vi "set_IMAQdxSession.vi"(3 "error in (no error)":errorcluster, 4 "IMAQdx Session":T1, 5 "HGF_ImaqDx in":refnum<class "HGF_ImaqDx.lvclass">) -> (0 "error out":errorcluster, 2 "HGF_ImaqDx out":refnum<class "HGF_ImaqDx.lvclass">)   [LabVIEW 2014, in "HGF_IMAQ.lvlib" / "HGF_ImaqDx.lvclass"]
doc: "Set member: IMAQdx Session."
uses:
  HGF_ImaqDx.lvclass
  <vilib>/userdefined/High Color/IMAQdx.ctl
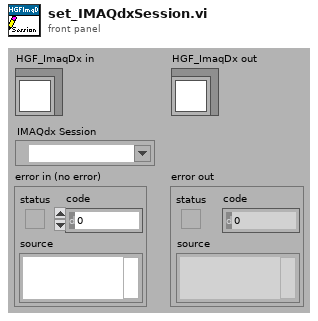
[diagram p1: front panel]
types:
  T1 = typedef "IMAQdx.ctl" = refnum<k21>
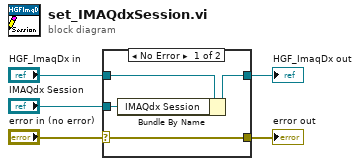
[diagram p0: block diagram]
diagram:
  n1 = case shown="No Error" "error in (no error)" {
    selector: "error in (no error)" -> [w9 w10]
    tunnel: [w9 w10] -> w4
    tunnel: [w7 w11] -> w2
    tunnel: "HGF_ImaqDx in" -> [w8 w11]
    tunnel: "IMAQdx Session" -> [w6 _]
    frame No Error {
      n2 = Bundle By Name(cluster=w8, "IMAQdx Session"=w6) -> (w7:refnum<class "HGF_ImaqDx.lvclass">)
    }
    frame Error {
    }
  }
  "error out" <- w4
  "HGF_ImaqDx out" <- w2
